vi "Deprecated Main.vi"() -> ()   [LabVIEW 2017]
uses:
  <vilib>/platform/TimedLoop/XDataNode/XDataNode.xnode
  <vilib>/Platform/TimedLoop/XDataNode/nitl_modes.ctl
  <vilib>/Platform/TimedLoop/XDataNode/XDNodeRunTimeDep.lvlib
  <vilib>/Platform/TimedLoop/XDataNode/wakeup.ctl
  <vilib>/Platform/TimedLoop/XDataNode/timing_clust.ctl
  <vilib>/Analysis/Matrix/Datatypes/RealMatrix.ctl
  <vilib>/Analysis/Matrix/NI_Matrix.lvlib
  <vilib>/Native 3D Graph/xcontrol/3DPC_SurfacePlot.xctl
  <vilib>/picture/3D Picture Control/NI_3D Picture Control.lvlib
  <vilib>/robotics/Kinematics/NI_Kinematics.lvlib
  <vilib>/picture/3D Picture Control/Object/Create Object (drawable).vi
  <vilib>/picture/3D Picture Control/Object/Add Object (no reference).vi
  <vilib>/Native 3D Graph/classes/Line/Line.lvclass
panel:
  out "v30":dbl[](array[numeric])=[0.09232183028825097, 0.47599704616100347, 0.8745876123626648]
  out "v20":dbl[](array[numeric])=[0.09232183028825097, 0.47599704616100347, 0.8745876123626648]
  out "v10":dbl[](array[numeric])=[0.09232183028825097, 0.47599704616100347, 0.8745876123626648]
  out "beta2":dbl=0.7460127831658563
  out "beta1":dbl=0.9553166181245091
  out "gamma2":dbl=1.2566370614359172
  out "gamma1":dbl=1.5707963267948966
  out "alpha2":dbl=1.5707963267948966
  out "alpha1":dbl=1.5707963267948966
  out "[thetad1 thetad2 thetad3]":dbl[](array[numeric])=[-0.20505895255510495, -0.3880041801893481, 0.5168516560729728]
  out "[thetac1 thetac2 thetac3]":dbl[](array[numeric])=[-0.20505895255510495, -0.3880041801893481, 0.5168516560729728]
  out "Rd":T1=[[0.999997873047629, -0.002062498537722336, 0.0], [0.002062498537722336, 0.999997873047629, 0.0], [0.0, 0.0, 1.0]]
  out "dt":dbl=0.001
  out "[vxc vyc omegac]":dbl[](array[numeric])=[-3141.5863074386834, -3141.5950633822936, -0.001813054229637956]
  out "[vxd vyd omegad]":dbl[](array[numeric])=[nan, nan, -514.7909691272001]
  out "[xc yc zc]":dbl[](array[numeric])=[2.936527354883579, 2.753590883192946, nan]
  out "[Fmx Fmy Tmz]":dbl[](array[numeric])=[nan, nan, 643.4864450912131]
  out "[xd yd phid]":dbl[](array[numeric])=[nan, nan, 0.0020625000000022986]
  out "[Fux Fuy Tuz]":dbl[](array[numeric])=[nan, nan, -643.4887114090002]
  out "3D Picture":refnum<vi>(3d-picture)
  out "3D Graph":refnum<class "Base Datatype.lvclass">[](xcontrol)
  in  "STOP":bool
  in  "Lever":dbl=1.0
  out "Period":i64=1
  out "[xc yc phic]":dbl[](array[numeric])=[-0.20505895255510495, -0.3880041801893481, 0.5168516560729728]
  out "Rc":T1=[[0.8693783298053238, -0.4941470627909323, 0.0], [0.4941470627909323, 0.8693783298053238, 0.0], [0.0, 0.0, 1.0]]
  out "[Fx Fy Tz]":dbl[](array[numeric])=[-0.0, 0.0, 0.0078125]
  in  "[Cx Cy Cz]":dbl[](array[numeric])=[1.25, 1.25, 1.25]
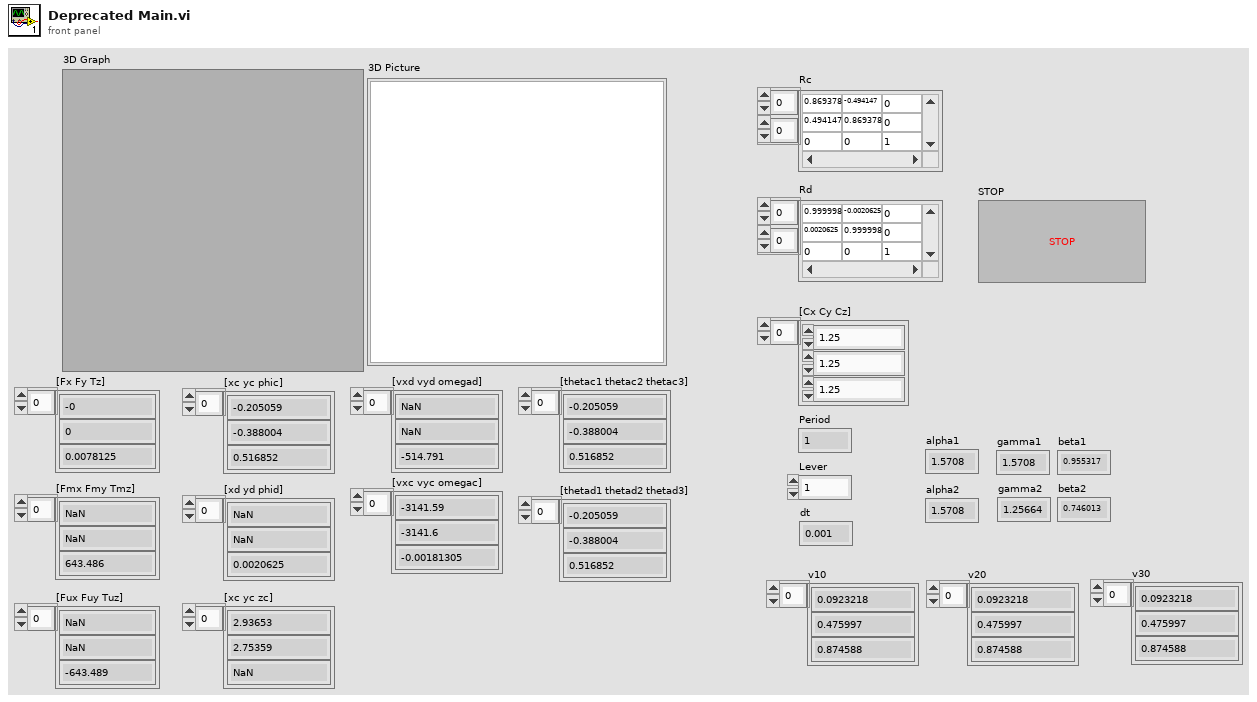
[diagram p1: front panel]
types:
  T1 = typedef "NI_Matrix.lvlib/RealMatrix.ctl" = dbl[][]
  T2 = typedef "XDNodeRunTimeDep.lvlib/timing_clust.ctl" = cluster{"Expected End [f-1]":u64, "Actual End [f-1]":u64, "Finished Late? [f-1]":bool, "Expected End [i-1]":u64, "Actual End [i-1]":u64, "Finished Late? [i-1]":bool, "Expected Start [i]":u64, "Actual Start [i]":u64, "Expected Start [f]":u64, "Actual Start [f]":u64, "Source Name":string, "Structure Name":string, "Period":i64, "Deadline":i64, "Offset":i64, "Start":i64, "Priority":i32, "Timeout":i32, "Mode":T3, "Wakeup Reason":T4, "Error":errorcluster, "Source Type":string, "Secondary Source Type":string, "Global End Time":u64, "Global Start Time":u64, "Frame Duration":u64, "Iteration Duration":u64, "Assigned CPU":i32, "I/O Scan Engine Mode":u32}
  T3 = typedef "XDNodeRunTimeDep.lvlib/nitl_modes.ctl" = enum32{"No Change", "Process missed periods, maintain original phase", "Discard missed periods, maintain original phase", "Process missed periods, ignore original phase", "Discard missed periods, ignore original phase"}
  T4 = typedef "XDNodeRunTimeDep.lvlib/wakeup.ctl" = enum32{"Normal", "Aborted", "Asynchronous wakeup", "Timing source error", "Timed loop error", "Timeout"}
  T5 = cluster{"vector[0]":dbl, "vector[1]":dbl, "vector[2]":dbl}
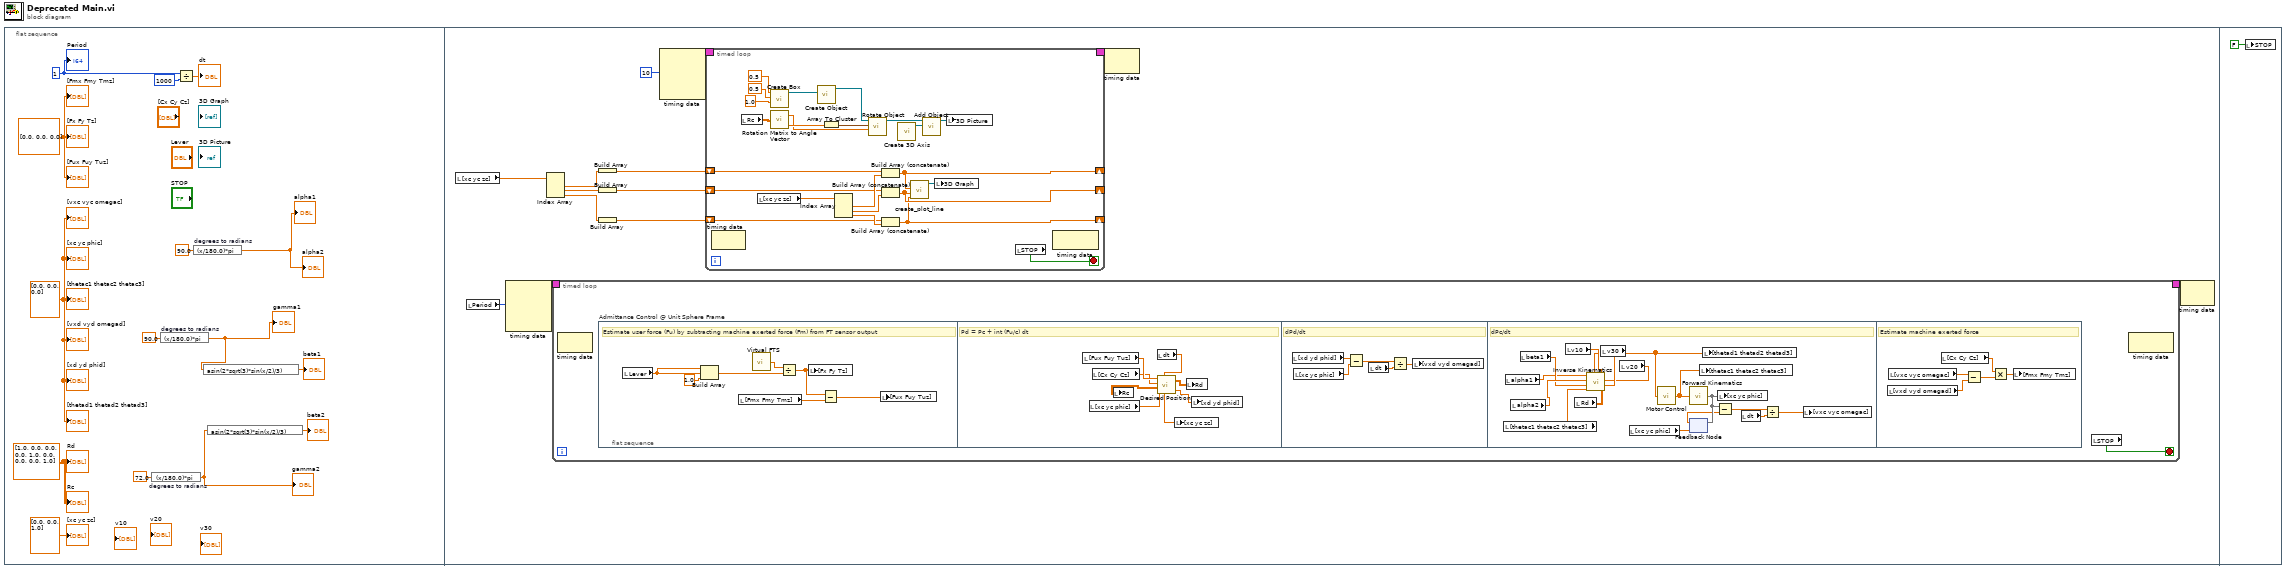
[diagram p0: block diagram]
diagram:
  n1 = flat-sequence {
    frame #0 {
      w13 = i64 1 ("Period")
      w15 = dbl[] [0.0, 0.0, 0.0] ("[Fx, Fy, Tz]")
      w9 = dbl[] [0.0, 0.0, 0.0] ("second subarray")
      w10 = T1 [[1.0, 0.0, 0.0], [0.0, 1.0, 0.0], [0.0, 0.0, 1.0]] ("calibration matrix 2")
      n2 = expression code="(x/180.0)*pi" "degrees to radians"(72.0) -> (w1:dbl)
      "gamma2" <- w1
      n3 = expression code="(x/180.0)*pi" "degrees to radians"(90.0) -> (w3:dbl)
      "gamma1" <- w3
      n4 = Divide(x=w13, y=i64 1000 ("Period")) -> (x/y=→"dt":dbl)
      n5 = expression code="(x/180.0)*pi" "degrees to radians"(90.0) -> (→"alpha1" →"alpha2":dbl)
      n6 = expression code="asin(2*sqrt(3)*sin(x/2)/3)"(w3) -> (→"beta1":dbl)
      n7 = expression code="asin(2*sqrt(3)*sin(x/2)/3)"(w1) -> (→"beta2":dbl)
      "[Fx Fy Tz]" <- w15
      "Rc" <- w10
      "[xc yc phic]" <- w9
      "Period" <- w13
      "[Fux Fuy Tuz]" <- w15
      "[xd yd phid]" <- w9
      "[Fmx Fmy Tmz]" <- w15
      "[xc yc zc]" <- dbl[] [0.0, 0.0, 1.0] ("second subarray")
      "[vxd vyd omegad]" <- w9
      "[vxc vyc omegac]" <- w9
      "Rd" <- w10
      "[thetad1 thetad2 thetad3]" <- w9
      "[thetac1 thetac2 thetac3]" <- w9
    }
    frame #1 {
      n8 = local read "[xc yc zc]"() -> (w16:dbl[])
      n9 = local read "Period"() -> (w23:i64)
      n10 = node-c288(w23) -> (w28:T2)  [unwired: 3 in]
      n11 = Index Array(array=w16) -> (element #1=w22:dbl, element #2=w20:dbl, element #3=w18:dbl)  [unwired: 3 in]
      n12 = timed-loop {
        timing: w28 -> [_]
        timing-out: [_] -> w27
        stop <- w59 stop-if-true
        n13 = node-c288() -> ()  [unwired: 1 in, 1 out]
        n14 = flat-sequence "Admittance Control @ Unit Sphere Frame" {
          frame #0 {
            # "Estimate user force (Fu) by subtracting machine exerted force (Fm) from FT sensor output"
            n15 = local read "Lever"() -> (w63:dbl)
            n16 = Build Array(w63, w63, 1.0 ("element")) -> (w61:dbl[])
            n17 = local read "[Fmx Fmy Tmz]"() -> (w66:dbl[])
            n18 = call "Virtual FTS.vi"() -> ("FT"=w60:dbl[])
            n19 = Divide(x=w60, y=w61) -> (x/y=w64:dbl[])
            n20 = local write "[Fx Fy Tz]"(w64) -> ()
            n21 = Subtract(x=w64, y=w66) -> (x-y=w65:dbl[])
            n22 = local write "[Fux Fuy Tuz]"(w65) -> ()
          }
          frame #1 {
            # "Pd = Pc + int (Fu/c) dt"
            n23 = local read "[Fux Fuy Tuz]"() -> (w74:dbl[])
            n24 = local read "[xc yc phic]"() -> (w71:dbl[])
            n25 = local read "[Cx Cy Cz]"() -> (w73:dbl[])
            n26 = local read "dt"() -> (w72:dbl)
            n27 = call "Desired Position.vi"("dt"=w72, "[xc yc phic]"=w71, "[Cx Cy Cz]"=w73, "[Fux Fuy Tuz]"=w74) -> ("[xd yd phid]"=w68:dbl[], "Rd"=w69:T1, "[xc yc zc]"=w67:dbl[], "Rc"=w70:T1)
            n28 = local write "Rc"(w70) -> ()
            n29 = local write "[xc yc zc]"(w67) -> ()
            n30 = local write "Rd"(w69) -> ()
            n31 = local write "[xd yd phid]"(w68) -> ()
          }
          frame #2 {
            # "dPd/dt"
            n32 = local read "[xd yd phid]"() -> (w79:dbl[])
            n33 = local read "[xc yc phic]"() -> (w78:dbl[])
            n34 = Subtract(x=w79, y=w78) -> (x-y=w77:dbl[])
            n35 = local read "dt"() -> (w75:dbl)
            n36 = Divide(x=w77, y=w75) -> (x/y=w76:dbl[])
            n37 = local write "[vxd vyd omegad]"(w76) -> ()
          }
          frame #3 {
            # "dPc/dt"
            n38 = local read "[thetac1 thetac2 thetac3]"() -> (w88:dbl[])
            n39 = local read "alpha1"() -> (w85:dbl)
            n40 = local read "alpha2"() -> (w87:dbl)
            n41 = local read "beta1"() -> (w86:dbl)
            n42 = local read "v10"() -> (w84:dbl[])
            n43 = local read "Rd"() -> (w89:T1)
            n44 = local read "v30"() -> (w83:dbl[])
            n45 = local read "v20"() -> (w82:dbl[])
            n46 = call "Inverse Kinematics.vi"("Rd"=w89, "v30"=w83, "v20"=w82, "v10"=w84, "[thetac1 thetac2 thetac3]"=w88, "beta1"=w86, "alpha2"=w87, "alpha1"=w85) -> ("[thetad1 thetad2 thetad3]"=w81:dbl[])
            n47 = local read "[xc yc phic]"() -> (w91:dbl[])
            n48 = call "Motor Control.vi"("[thetad1 thetad2 thetad3]"=w81) -> ("[thetac1 thetac2 thetac3]"=w80:dbl[])
            n49 = call "Forward Kinematics.vi"("[thetac1 thetac2 thetac3]"=w80) -> (0:w93)
            n50 = feedback #1(w91) -> (w92:dbl[])
            n51 = feedback-in #1(w93) -> ()
            n52 = local write "[thetac1 thetac2 thetac3]"(w80) -> ()
            n53 = local write "[thetad1 thetad2 thetad3]"(w81) -> ()
            n54 = Subtract(x=w93, y=w92) -> (x-y=w95:dbl[])
            n55 = local write "[xc yc phic]"(w93) -> ()
            n56 = local read "dt"() -> (w90:dbl)
            n57 = Divide(x=w95, y=w90) -> (x/y=w94:dbl[])
            n58 = local write "[vxc vyc omegac]"(w94) -> ()
          }
          frame #4 {
            # "Estimate machine exerted force"
            n59 = local read "[vxd vyd omegad]"() -> (w99:dbl[])
            n60 = local read "[vxc vyc omegac]"() -> (w100:dbl[])
            n61 = local read "[Cx Cy Cz]"() -> (w97:dbl[])
            n62 = Subtract(x=w100, y=w99) -> (x-y=w98:dbl[])
            n63 = Multiply(x=w97, y=w98) -> (x*y=w96:dbl[])
            n64 = local write "[Fmx Fmy Tmz]"(w96) -> ()
          }
        }
        n65 = local read "STOP"() -> (w59:bool)
        n66 = node-c288() -> ()  [unwired: 1 in, 1 out]
      }
      n67 = Build Array(w22) -> (w21:dbl[])
      n68 = Build Array(w20) -> (w19:dbl[])
      n69 = Build Array(w18) -> (w17:dbl[])
      n70 = node-c288(i64 10 ("Period")) -> (w26:T2)  [unwired: 3 in]
      n71 = timed-loop {
        timing: w26 -> [_]
        timing-out: [_] -> w25
        shift-right: [w46] -> _
        shift-left: w21 -> [w47]
        shift-right: [w44] -> _
        shift-left: w19 -> [w45]
        shift-right: [w41] -> _
        shift-left: w17 -> [w42]
        stop <- w51 stop-if-true
        n72 = node-c288() -> ()  [unwired: 1 in, 1 out]
        n73 = local read "Rc"() -> (w40:T1)
        n74 = local read "[xc yc zc]"() -> (w52:dbl[])
        n75 = call <vilib>:"Create Box.vi"("Length Z"=sgl 1.0, "Length Y"=sgl 0.5, "Length X"=sgl 0.5) -> ("New Box Refnum"=w33:refnum<vi>)  [unwired: 7 in, 1 out]
        n76 = call <vilib>:"Rotation Matrix to Angle Vector.vi"("rotation matrix"=w40) -> ("angle"=w36:dbl, "vector"=w39:dbl[])
        n77 = call-poly <vilib>:"Create Object.vi"("Geometry"=w33) -> ("Scene:New Object"=w30:refnum<vi>)  [unwired: 9 in, 1 out]
        n78 = Array To Cluster(array=w39) -> (cluster=w37:T5)
        n79 = Index Array(array=w52) -> (element #1=w50:dbl, element #2=w49:dbl, element #3=w48:dbl)  [unwired: 3 in]
        n80 = call <vilib>:"Rotate Object.vi"("Angle"=w36, "Axis"=w37, "Scene.Object In"=w30) -> ("Scene.Object Out"=w35:refnum<vi>)  [unwired: 7 in, 1 out]
        n81 = Build Array (concatenate)(w47, w50) -> (w46:dbl[])
        n82 = Build Array (concatenate)(w45, w49) -> (w44:dbl[])
        n83 = Build Array (concatenate)(w42, w48) -> (w41:dbl[])
        n84 = call <vilib>:"Create 3D Axis.vi"() -> ("New Object Refnum"=w29:refnum<vi>)  [unwired: 10 in, 1 out]
        n85 = call <vilib>:"create_plot_line.vi"("z vector"=w41, "y vector"=w44, "x vector"=w46) -> ("plots out"=w43:refnum<class "Base Datatype.lvclass">[])  [unwired: 2 in, 6 out]
        n86 = call-poly <vilib>:"Add Object.vi"("New Object In"=w29, "Scene Object In"=w35) -> ("Scene Object Out"=w38:refnum<vi>)  [unwired: 8 in, 1 out]
        n87 = local write "3D Graph"(w43) -> ()
        n88 = local write "3D Picture"(w38) -> ()
        n89 = local read "STOP"() -> (w51:bool)
        n90 = node-c288() -> ()  [unwired: 1 in, 1 out]
      }
      n91 = node-c288(w25) -> ()  [unwired: 1 out]
      n92 = node-c288(w27) -> ()  [unwired: 1 out]
    }
    frame #2 {
      n93 = local write "STOP"(FALSE ("STOP")) -> ()
    }
  }
